vi "Configure Trigger Alarm.vi"(5 "RepeatCount":i32 format="%.0g", 6 "Period":dbl, 7 "TimeFraction":dbl, 8 "error in (no error)":errorcluster {"code" format="%.0x"}, 9 "TimeSeconds":dbl, 10 "AlarmName":string="ALARM0" caption="AlarmName (ALARM0)", 11 "instrument handle":refnum<k15>) -> (0 "error out":errorcluster {"code" format="%.0x"}, 3 "instrument handle out":refnum<k15>)   [LabVIEW 2009, in "Keysight XSAn.lvlib"]
doc: "This VI configures the most commonly configured properties of the trigger alarm sub-system.\n\nSupported Models: N9000A, N9000B, N9010A, N9010B, N9020A, N9020B, N9030A, N9030B, N9038A, SPN9003A, SPN9026A"
uses:
  <instrlib>/Keysight XSAn/Keysight XSAn.lvlib
  AgXSAn.dll
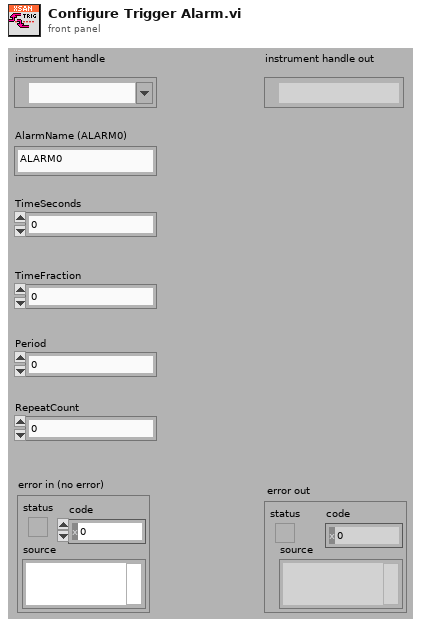
[diagram p1: front panel]
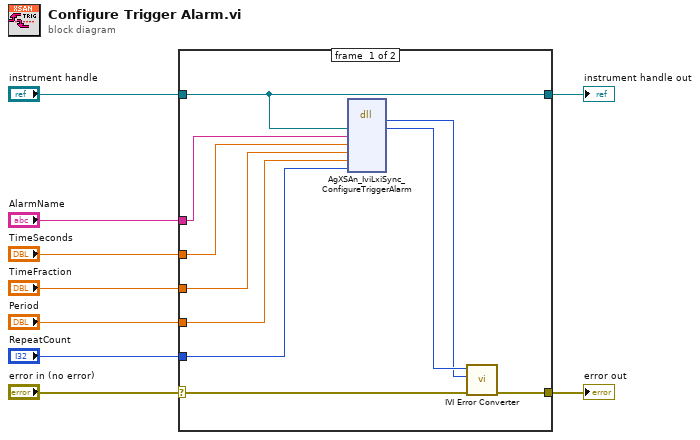
[diagram p0: block diagram]
diagram:
  n1 = case shown="No Error" "error in (no error)" {
    selector: "error in (no error)" -> [w17 w21]
    tunnel: [w16 w21] -> w9
    tunnel: "instrument handle" -> [w10 w20]
    tunnel: "AlarmName" -> [w15 _]
    tunnel: "TimeSeconds" -> [w14 _]
    tunnel: "TimeFraction" -> [w13 _]
    tunnel: "Period" -> [w12 _]
    tunnel: "RepeatCount" -> [w11 _]
    tunnel: [w10 w20] -> w1
    frame #0 {
      n2 = dll-call lib="AgXSAn**.dll" fn="AgXSAn_IviLxiSync_ConfigureTriggerAlarm"("Vi"=w10, "AlarmName"=w15, "TimeSeconds"=w14, "TimeFraction"=w13, "Period"=w12, "RepeatCount"=w11) -> (w18:i32, "Vi"=w19:u32)  [unwired: 8 in, 2 out]
      n3 = call <instrlib>:"IVI Error Converter.vi"("error in (no error)"=w17, "IVI error code (0)"=w18, "instrument handle"=w19) -> ("error out"=w16:errorcluster)  [unwired: 7 in, 1 out]
    }
    frame #1 {
    }
  }
  "error out" <- w9
  "instrument handle out" <- w1
